vi "Test.vi"(8 "error in (no error)":errorcluster, 11 "Another Concrete Step in":refnum<class "Another Concrete Step.lvclass">) -> (0 "error out":errorcluster, 2 "Pass?":bool, 3 "Another Concrete Step out":refnum<class "Another Concrete Step.lvclass">)   [LabVIEW 2020, in "Another Concrete Step.lvclass"]
uses:
  Another Concrete Step.lvclass
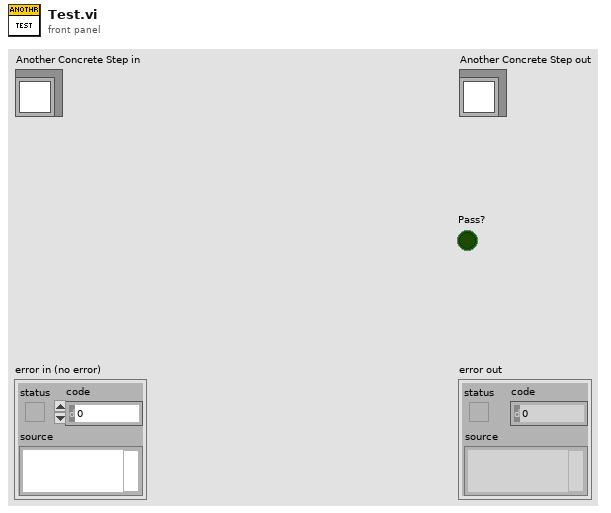
[diagram p1: front panel]
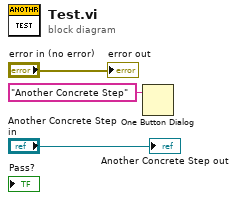
[diagram p0: block diagram]
diagram:
  n1 = One Button Dialog(message="Another Concrete Step") -> ()  [unwired: 1 in, 1 out]
  "error out" <- "error in (no error)"
  "Another Concrete Step out" <- "Another Concrete Step in"
